vi "Windows虚拟键盘调用.vi"(8 "error in (no error)":errorcluster caption="错误输入（无错误）") -> (0 "error out":errorcluster caption="错误输出")   [LabVIEW 2018]
uses:
  kernel32.dll
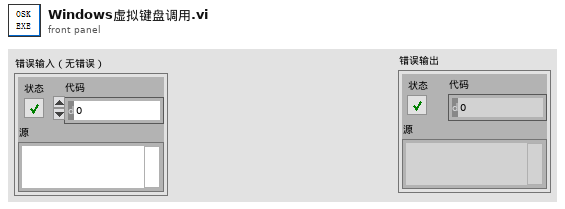
[diagram p1: front panel]
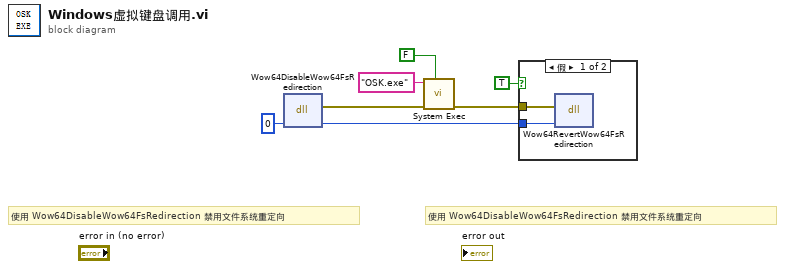
[diagram p0: block diagram]
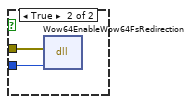
[diagram p2: hidden frame]
diagram:
  # "使用 Wow64DisableWow64FsRedirection 禁用文件系统重定向"
  # "使用 Wow64DisableWow64FsRedirection 禁用文件系统重定向"
  n1 = dll-call lib="kernel32.dll" fn="Wow64DisableWow64FsRedirection"("OldValue"=0) -> (error out=w5:errorcluster, "OldValue"=w2:i32)  [unwired: 4 in, 1 out]
  n2 = call <vilib>:"System Exec.vi"("wait until completion? (T)"=FALSE, "error in (no error)"=w5, "command line"="OSK.exe") -> ("error out"=w4:errorcluster)  [unwired: 5 in, 3 out]
  n3 = case shown="假" TRUE {
    tunnel: w4 -> [w9 w11]
    tunnel: w2 -> [w8 w10]
    frame False {
      n4 = dll-call lib="kernel32.dll" fn="Wow64RevertWow64FsRedirection"(error in=w9, "OldValue"=w8) -> ()  [unwired: 4 in, 2 out]
    }
    frame True {
      n5 = dll-call lib="kernel32.dll" fn="Wow64EnableWow64FsRedirection"(error in=w11, "OldValue"=w10) -> ()  [unwired: 4 in, 2 out]
    }
  }
